vi "main.vi"() -> ()   [LabVIEW 2010]
uses:
  common/xcontrols/XImage/XImage/XImage.xctl
  common/classes/ImageCollection/ImageCollection/ImageCollection.lvclass
  common/classes/PointCollection/PointCollection/PointCollection.lvclass
panel:
  in  "buttonExportB":bool
  in  "buttonExportA":bool
  in  "Tab Control":enum32{"Rotation fitting"}(tab)
  out "translation vector":dbl[](array[numeric])
  out "rotation fit angles":dbl[unit][](array[numeric])
  out "scale factor":dbl
  in  "buttonRotFit":bool
  in  "increment step":dbl[unit]=0.017453292519943295
  in  "buttonStop":bool
  in  "Image stack B":refnum<class "ImageCollection.lvclass">(xcontrol)
  in  "Image stack A":refnum<class "ImageCollection.lvclass">(xcontrol)
  # "CellMatcher"
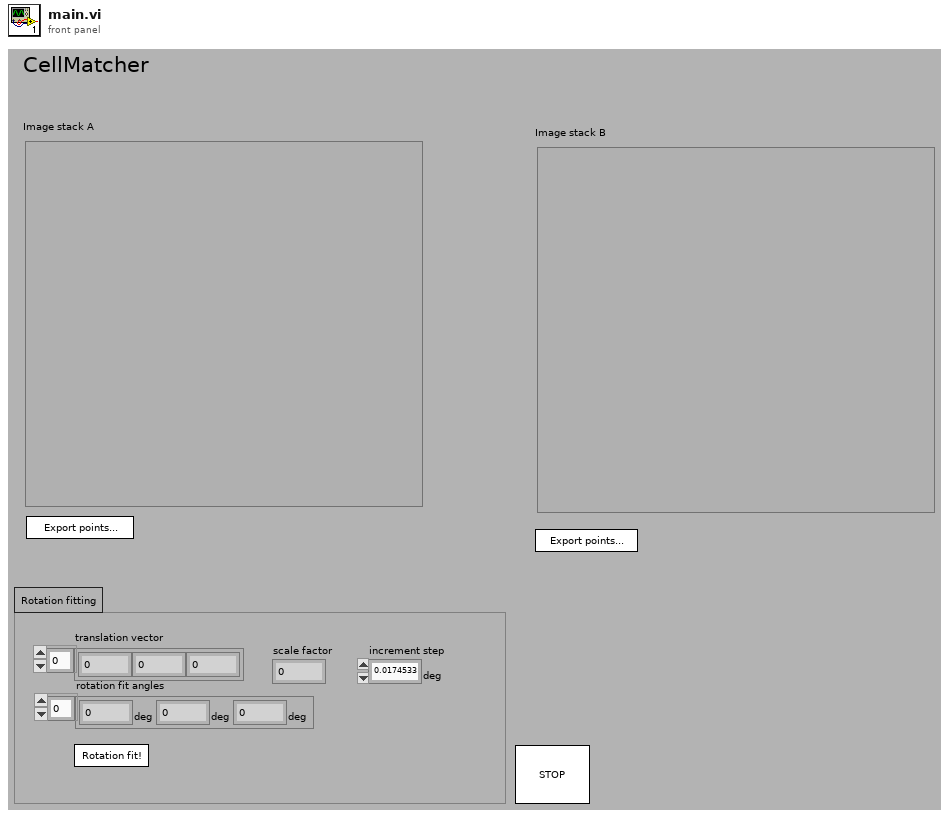
[diagram p1: front panel]
types:
  T1 = cluster{"PointCollection.lvclass":refnum<class "PointCollection.lvclass">, "PointCollection.lvclass":refnum<class "PointCollection.lvclass">}
  T2 = cluster{"[0]":refnum<class "PointCollection.lvclass">, "[1]":refnum<class "PointCollection.lvclass">}
  T3 = cluster{"Global Rectangle":i32[], "Contours":cluster{"Contour Type":u32, "ROI Type":u32, "Points":i32[]}[]}[]
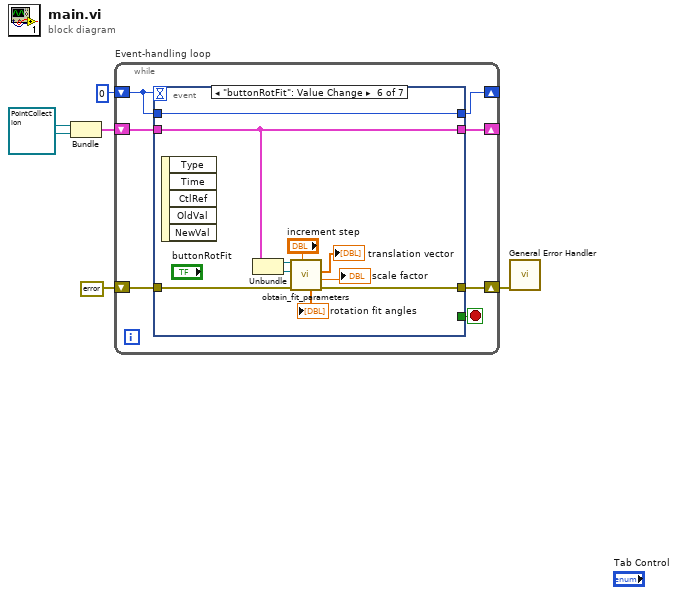
[diagram p0: block diagram]
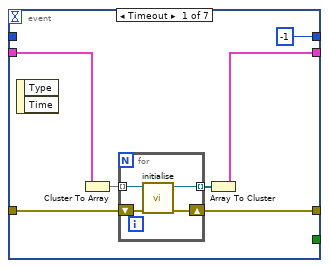
[diagram p2: hidden frame]
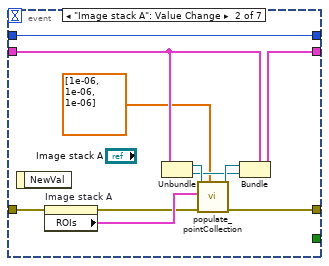
[diagram p3: hidden frame]
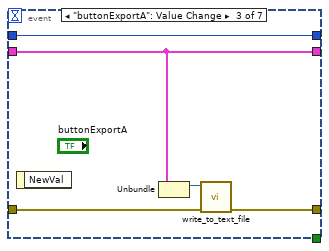
[diagram p4: hidden frame]
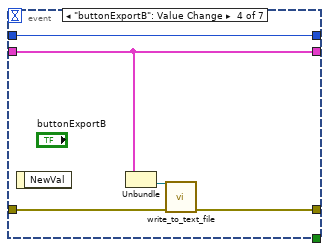
[diagram p5: hidden frame]
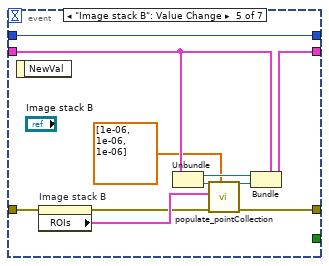
[diagram p6: hidden frame]
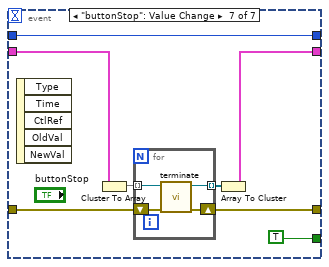
[diagram p7: hidden frame]
diagram:
  w2 = refnum<class "PointCollection.lvclass"> refnum ("PointCollection.lvclass")
  n1 = Bundle("PointCollection.lvclass"=w2, "PointCollection.lvclass"=w2) -> (w3:T1)  [unwired: 1 in]
  n2 = while "Event-handling loop" {
    shift-right: [w11] -> w4
    shift-left: errorcluster {"status"=FALSE, "code"=0, "source"=""} ("error in (no error)") -> [w12]
    shift-right: [w8] -> _
    shift-left: w3 -> [w9]
    shift-right: [w6] -> _
    shift-left: 0 -> [w7]
    stop <- w10 stop-if-true
    n3 = event shown="[5] \"buttonRotFit\": Value Change" {
      selector: _ -> [_ _ _ _ _ _ _]
      dyn-events: _ -> [_ _ _ _ _ _ _]
      timeout: w7 -> [_ _ _ _ _ _ _]
      tunnel: w12 -> [w18 w33 w36 w43 w54 w64 w71]
      tunnel: [w17 w32 w35 w42 w53 w63 w70] -> w11
      tunnel: [_ _ _ _ _ _ TRUE] -> w10
      tunnel: w9 -> [w14 w31 w38 w41 w50 w62 w67]
      tunnel: [w13 w30 w38 w41 w49 w62 w66] -> w8
      tunnel: [-1 w34 w39 w44 w55 w65 w72] -> w6
      tunnel: w7 -> [_ w34 w39 w44 w55 w65 w72]
      event Timeout {
        n4 = event-data() -> ()  [unwired: 1 in, 2 out]
        n5 = Cluster To Array(cluster=w14) -> (array=w16:refnum<class "PointCollection.lvclass">[])
        n6 = for {
          shift-right: [w22] -> w17
          shift-left: w18 -> [w23]
          tunnel: w16 -> [w21] mode=indexing
          tunnel: [w20] -> w15 mode=indexing
          n7 = call "initialise.vi"("error in (no error)"=w23, "PointCollection in"=w21) -> ("error out"=w22:errorcluster, "PointCollection out"=w20:refnum<class "PointCollection.lvclass">)  [unwired: 8 in]
        }
        n8 = Array To Cluster(array=w15) -> (cluster=w13:T2)
      }
      event "Image stack A": Value Change {
        n9 = event-data() -> ()  [unwired: 1 in, 1 out]
        n10 = property on="Image stack A" class="XImage (strict)"(error in=w33) -> (error out=w25:errorcluster, "ROIs"=w26:T3)  [unwired: 1 in, 1 out]
        n11 = Unbundle(w31) -> ("PointCollection.lvclass"=w29:refnum<class "PointCollection.lvclass">, "PointCollection.lvclass"=w27:refnum<class "PointCollection.lvclass">)
        n12 = call "populate_pointCollection.vi"("calibration"=dbl[unit][] [1e-06, 1e-06, 1e-06], "error in (no error)"=w25, "ROI:ROIs"=w26, "PointCollection.lvclass in"=w29) -> ("error out"=w32:errorcluster, "PointCollection.lvclass out"=w28:refnum<class "PointCollection.lvclass">)  [unwired: 6 in]
        n13 = Bundle(cluster=w31, "PointCollection.lvclass"=w28, "PointCollection.lvclass"=w27) -> (w30:T1)
      }
      event "buttonExportA": Value Change {
        n14 = event-data() -> ()  [unwired: 1 in, 1 out]
        n15 = Unbundle(w38) -> ("PointCollection.lvclass"=w37:refnum<class "PointCollection.lvclass">)  [unwired: 1 out]
        n16 = call "write_to_text_file.vi"("error in (no error)"=w36, "PointCollection in"=w37) -> ("error out"=w35:errorcluster)  [unwired: 8 in, 1 out]
      }
      event "buttonExportB": Value Change {
        n17 = event-data() -> ()  [unwired: 1 in, 1 out]
        n18 = Unbundle(w41) -> ("PointCollection.lvclass"=w40:refnum<class "PointCollection.lvclass">)  [unwired: 1 out]
        n19 = call "write_to_text_file.vi"("error in (no error)"=w43, "PointCollection in"=w40) -> ("error out"=w42:errorcluster)  [unwired: 8 in, 1 out]
      }
      event "Image stack B": Value Change {
        n20 = event-data() -> ()  [unwired: 1 in, 1 out]
        n21 = property on="Image stack B" class="XImage (strict)"(error in=w54) -> (error out=w46:errorcluster, "ROIs"=w47:T3)  [unwired: 1 in, 1 out]
        n22 = Unbundle(w50) -> ("PointCollection.lvclass"=w51:refnum<class "PointCollection.lvclass">, "PointCollection.lvclass"=w52:refnum<class "PointCollection.lvclass">)
        n23 = call "populate_pointCollection.vi"("calibration"=dbl[unit][] [1e-06, 1e-06, 1e-06], "error in (no error)"=w46, "ROI:ROIs"=w47, "PointCollection.lvclass in"=w52) -> ("error out"=w53:errorcluster, "PointCollection.lvclass out"=w48:refnum<class "PointCollection.lvclass">)  [unwired: 6 in]
        n24 = Bundle(cluster=w50, "PointCollection.lvclass"=w51, "PointCollection.lvclass"=w48) -> (w49:T1)
      }
      event "buttonRotFit": Value Change {
        n25 = event-data() -> ()  [unwired: 1 in, 5 out]
        n26 = Unbundle(w62) -> ("PointCollection.lvclass"=w61:refnum<class "PointCollection.lvclass">, "PointCollection.lvclass"=w60:refnum<class "PointCollection.lvclass">)
        n27 = call-dynamic "obtain_fit_parameters.vi"("increment step"="increment step", "error in (no error)"=w64, "PointCollection B"=w60, "PointCollection in"=w61) -> ("error out"=w63:errorcluster, "scale factor"=→"scale factor":dbl, "translation vector"=→"translation vector":dbl[], "rotation fit angles"=→"rotation fit angles":dbl[unit][])  [unwired: 3 in, 1 out]
      }
      event "buttonStop": Value Change {
        n28 = event-data() -> ()  [unwired: 1 in, 5 out]
        n29 = Cluster To Array(cluster=w67) -> (array=w69:refnum<class "PointCollection.lvclass">[])
        n30 = for {
          shift-right: [w76] -> w70
          shift-left: w71 -> [w77]
          tunnel: w69 -> [w75] mode=indexing
          tunnel: [w74] -> w68 mode=indexing
          n31 = call-dynamic "terminate.vi"("error in (no error)"=w77, "PointCollection in"=w75) -> ("error out"=w76:errorcluster, "PointCollection out"=w74:refnum<class "PointCollection.lvclass">)  [unwired: 7 in, 1 out]
        }
        n32 = Array To Cluster(array=w68) -> (cluster=w66:T2)
      }
    }
  }
  n33 = call <vilib>:"General Error Handler.vi"("error in (no error)"=w4) -> ()  [unwired: 10 in, 5 out]
